vi "Evaluate Fitness.vi"(8 "error in":errorcluster, 10 "IChromosome Target in":refnum<class "IChromosome.lvclass">, 11 "IChromosome in":refnum<class "IChromosome.lvclass">) -> (0 "error out":errorcluster, 3 "IChromosome out":refnum<class "IChromosome.lvclass">)   [LabVIEW 2016, in "IChromosome.lvclass"]
uses:
  IChromosome.lvclass
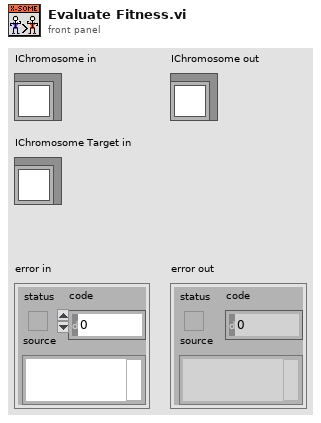
[diagram p1: front panel]
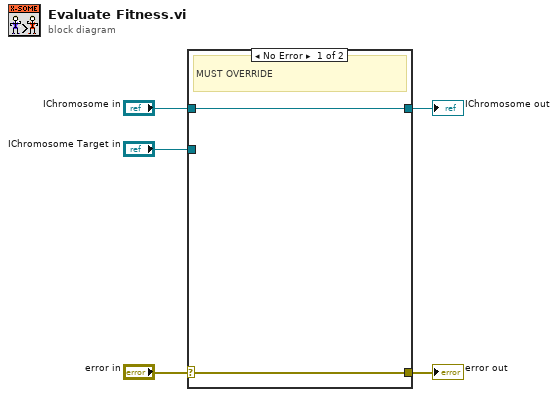
[diagram p0: block diagram]
diagram:
  n1 = case shown="No Error" "error in" {
    selector: "error in" -> [w7 w9]
    tunnel: [w7 w9] -> w4
    tunnel: [w6 w8] -> w2
    tunnel: "IChromosome in" -> [w6 w8]
    tunnel: "IChromosome Target in" -> [_ _]
    frame No Error {
      # "MUST OVERRIDE"
    }
    frame Error {
      # "MUST OVERRIDE"
    }
  }
  "error out" <- w4
  "IChromosome out" <- w2
